vi "HOST.vi"() -> ()   [LabVIEW 2018]
uses:
  <vilib>/userdefined/High Color/nirio_resource_hc.ctl
  <vilib>/FPGAPlugInAG/PXI-7953R/niLvFpga_Open_PXI-7953R.vi
  <vilib>/rvi/interface/common/dynamic/niFpgaDynamicAddResources.vi
  <vilib>/FPGAPlugInAG/Dynamic/niLvFpga_Reset_Dynamic.vi
  <vilib>/FPGAPlugInAG/Dynamic/niLvFpga_Run_Dynamic.vi
  <vilib>/FPGAPlugInAG/PXI-7841R/niLvFpga_Open_PXI-7841R.vi
  <vilib>/Utility/error.llb/Error Cluster From Error Code.vi
  <vilib>/rvi/errors/niLvFpgaAdjustHostInterfaceError.vi
  <vilib>/rvi/interface/nirviOpenFPGA/nirviOpenFPGA.xnode
  FPGA Bitfiles/Testfor6581_FPGATarget_Testfor6581_omxlOdkNot8.lvbitx
  <vilib>/rvi/interface/nirviMethod/nirviMethod.xnode
  FPGA Bitfiles/Testfor65817841_FPGATarget2_Testfor7841_mCGf3KCUrBc.lvbitx
  <vilib>/rvi/interface/nirviReadWriteControl/nirviReadWriteControl.xnode
  NiFpgaLv.dll
  <vilib>/rvi/interface/Simulation/niFpgaSimulationCallBeginRW.vi
panel:
  in  "Connector0/DIO15":bool
  in  "Connector0/DIO14":bool
  in  "Connector0/DIO13":bool
  in  "Connector0/DIO12":bool
  in  "Connector0/DIO11":bool
  in  "Connector0/DIO10":bool
  in  "Connector0/DIO9":bool
  in  "Connector0/DIO8":bool
  in  "Connector0/DIO7":bool
  in  "Connector0/DIO6":bool
  in  "Connector0/DIO5":bool
  in  "Connector0/DIO4":bool
  in  "Connector1/DIO15":bool
  in  "Connector0/DIO3":bool
  in  "Connector0/DIO2":bool
  in  "Connector0/DIO1":bool
  in  "Connector0/DIO0":bool
  in  "Connector2/DIO0":bool
  in  "Connector2/DIO1":bool
  in  "Connector2/DIO2":bool
  in  "Connector2/DIO3":bool
  in  "Connector2/DIO4":bool
  in  "Connector2/DIO5":bool
  in  "Connector2/DIO6":bool
  in  "Connector2/DIO7":bool
  in  "Connector2/DIO8":bool
  in  "Connector2/DIO9":bool
  in  "Connector2/DIO10":bool
  in  "Connector2/DIO11":bool
  in  "Connector2/DIO12":bool
  in  "Connector2/DIO13":bool
  in  "Connector2/DIO14":bool
  in  "Connector2/DIO15":bool
  in  "Connector2/DIO16":bool
  in  "Connector2/DIO17":bool
  in  "Connector2/DIO18":bool
  in  "Connector2/DIO19":bool
  in  "Connector2/DIO20":bool
  in  "Connector2/DIO21":bool
  in  "Connector2/DIO22":bool
  in  "Connector2/DIO23":bool
  in  "Connector2/DIO24":bool
  in  "Connector2/DIO25":bool
  in  "Connector2/DIO26":bool
  in  "Connector2/DIO27":bool
  in  "Connector2/DIO28":bool
  in  "Connector2/DIO29":bool
  in  "Connector2/DIO30":bool
  in  "Connector2/DIO31":bool
  in  "Connector2/DIO32":bool
  in  "Connector2/DIO33":bool
  in  "Connector2/DIO34":bool
  in  "Connector2/DIO35":bool
  in  "Connector2/DIO36":bool
  in  "Connector2/DIO37":bool
  in  "Connector2/DIO38":bool
  in  "Connector2/DIO39":bool
  in  "Connector1/DIO39":bool
  in  "Connector1/DIO38":bool
  in  "Connector1/DIO37":bool
  in  "Connector1/DIO36":bool
  in  "Connector1/DIO35":bool
  in  "Connector1/DIO34":bool
  in  "Connector1/DIO33":bool
  in  "Connector1/DIO32":bool
  in  "Connector1/DIO31":bool
  in  "Connector1/DIO30":bool
  in  "Connector1/DIO29":bool
  in  "Connector1/DIO28":bool
  in  "Connector1/DIO27":bool
  in  "Connector1/DIO26":bool
  in  "Connector1/DIO25":bool
  in  "Connector1/DIO24":bool
  in  "Connector1/DIO23":bool
  in  "Connector1/DIO22":bool
  in  "Connector1/DIO21":bool
  in  "Connector1/DIO20":bool
  in  "Connector1/DIO19":bool
  in  "Connector1/DIO18":bool
  in  "Connector1/DIO17":bool
  in  "Connector1/DIO16":bool
  in  "Connector1/DIO14":bool
  in  "Connector1/DIO13":bool
  in  "Connector1/DIO12":bool
  in  "Connector1/DIO11":bool
  in  "Connector1/DIO10":bool
  in  "Connector1/DIO9":bool
  in  "Connector1/DIO8":bool
  in  "Connector1/DIO7":bool
  in  "Connector1/DIO6":bool
  in  "Connector1/DIO5":bool
  in  "Connector1/DIO4":bool
  in  "Connector1/DIO3":bool
  in  "Connector1/DIO2":bool
  in  "Connector1/DIO1":bool
  in  "Connector1/DIO0":bool
  out "Connector0/AI7":i16
  out "Connector0/AI6":i16
  out "Connector0/AI5":i16
  out "Connector0/AI4":i16
  out "Connector0/AI3":i16
  out "Connector0/AI2":i16
  out "Connector0/AI1":i16
  out "Connector0/AI0":i16
  in  "Connector0/AO7":i16
  in  "Connector0/AO6":i16
  in  "Connector0/AO5":i16
  in  "Connector0/AO4":i16
  in  "Connector0/AO3":i16
  in  "Connector0/AO2":i16
  in  "Connector0/AO1":i16
  in  "Connector0/AO0":i16
  in  "Tab Control":enum32{"7953", "7841"}(tab)
  in  "IO Module\\DDCA_DIO0_Write":bool
  in  "IO Module\\DDCA_DIO1_Write":bool
  in  "IO Module\\DDCA_DIO2_Write":bool
  in  "IO Module\\DDCA_DIO3_Write":bool
  in  "IO Module\\DDCA_DIO4_Write":bool
  in  "IO Module\\DDCA_DIO5_Write":bool
  in  "IO Module\\DDCA_DIO6_Write":bool
  in  "IO Module\\DDCA_DIO7_Write":bool
  in  "IO Module\\DDCA_DIO8_Write":bool
  in  "IO Module\\DDCA_DIO9_Write":bool
  in  "IO Module\\DDCA_DIO10_Write":bool
  in  "IO Module\\DDCA_DIO11_Write":bool
  in  "IO Module\\DDCA_DIO12_Write":bool
  in  "IO Module\\DDCA_DIO13_Write":bool
  in  "IO Module\\DDCA_DIO14_Write":bool
  in  "IO Module\\DDCA_DIO15_Write":bool
  in  "IO Module\\DDCA_DIO16_Write":bool
  in  "IO Module\\DDCA_DIO17_Write":bool
  in  "IO Module\\DDCA_DIO18_Write":bool
  in  "IO Module\\DDCA_DIO19_Write":bool
  in  "IO Module\\DDCA_DIO20_Write":bool
  in  "IO Module\\DDCA_DIO21_Write":bool
  in  "IO Module\\DDCA_DIO22_Write":bool
  in  "IO Module\\DDCA_DIO23_Write":bool
  in  "IO Module\\DDCA_PFI1_Write":bool
  in  "IO Module\\DDCA_PFI2_Write":bool
  in  "IO Module\\DDCA_PFI3_Write":bool
  in  "IO Module\\DDCB_DIO0_Write":bool
  in  "IO Module\\DDCB_DIO1_Write":bool
  in  "IO Module\\DDCB_DIO2_Write":bool
  in  "IO Module\\DDCB_DIO3_Write":bool
  in  "IO Module\\DDCB_DIO4_Write":bool
  in  "IO Module\\DDCB_DIO5_Write":bool
  in  "IO Module\\DDCB_DIO6_Write":bool
  in  "IO Module\\DDCB_DIO7_Write":bool
  in  "IO Module\\DDCB_DIO8_Write":bool
  in  "IO Module\\DDCB_DIO9_Write":bool
  in  "IO Module\\DDCB_DIO10_Write":bool
  in  "IO Module\\DDCB_DIO11_Write":bool
  in  "IO Module\\DDCB_DIO12_Write":bool
  in  "IO Module\\DDCB_DIO13_Write":bool
  in  "IO Module\\DDCB_DIO14_Write":bool
  in  "IO Module\\DDCB_DIO15_Write":bool
  in  "IO Module\\DDCB_DIO16_Write":bool
  in  "IO Module\\DDCB_DIO17_Write":bool
  in  "IO Module\\DDCB_DIO18_Write":bool
  in  "IO Module\\DDCB_DIO19_Write":bool
  in  "IO Module\\DDCB_DIO20_Write":bool
  in  "IO Module\\DDCB_DIO21_Write":bool
  in  "IO Module\\DDCB_DIO22_Write":bool
  in  "IO Module\\DDCB_DIO23_Write":bool
  in  "IO Module\\DDCB_PFI1_Write":bool
  in  "IO Module\\DDCB_PFI2_Write":bool
  in  "IO Module\\DDCB_PFI3_Write":bool
  in  "7841":T1="PXI1Slot6"
  in  "Devider Frequency 160/(x*2), x>0":u8=1 min=1
  in  "Constant(F) / Frequency(T)":bool
  in  "Стоп":bool
  in  "7953R":T1="PXI1Slot6"
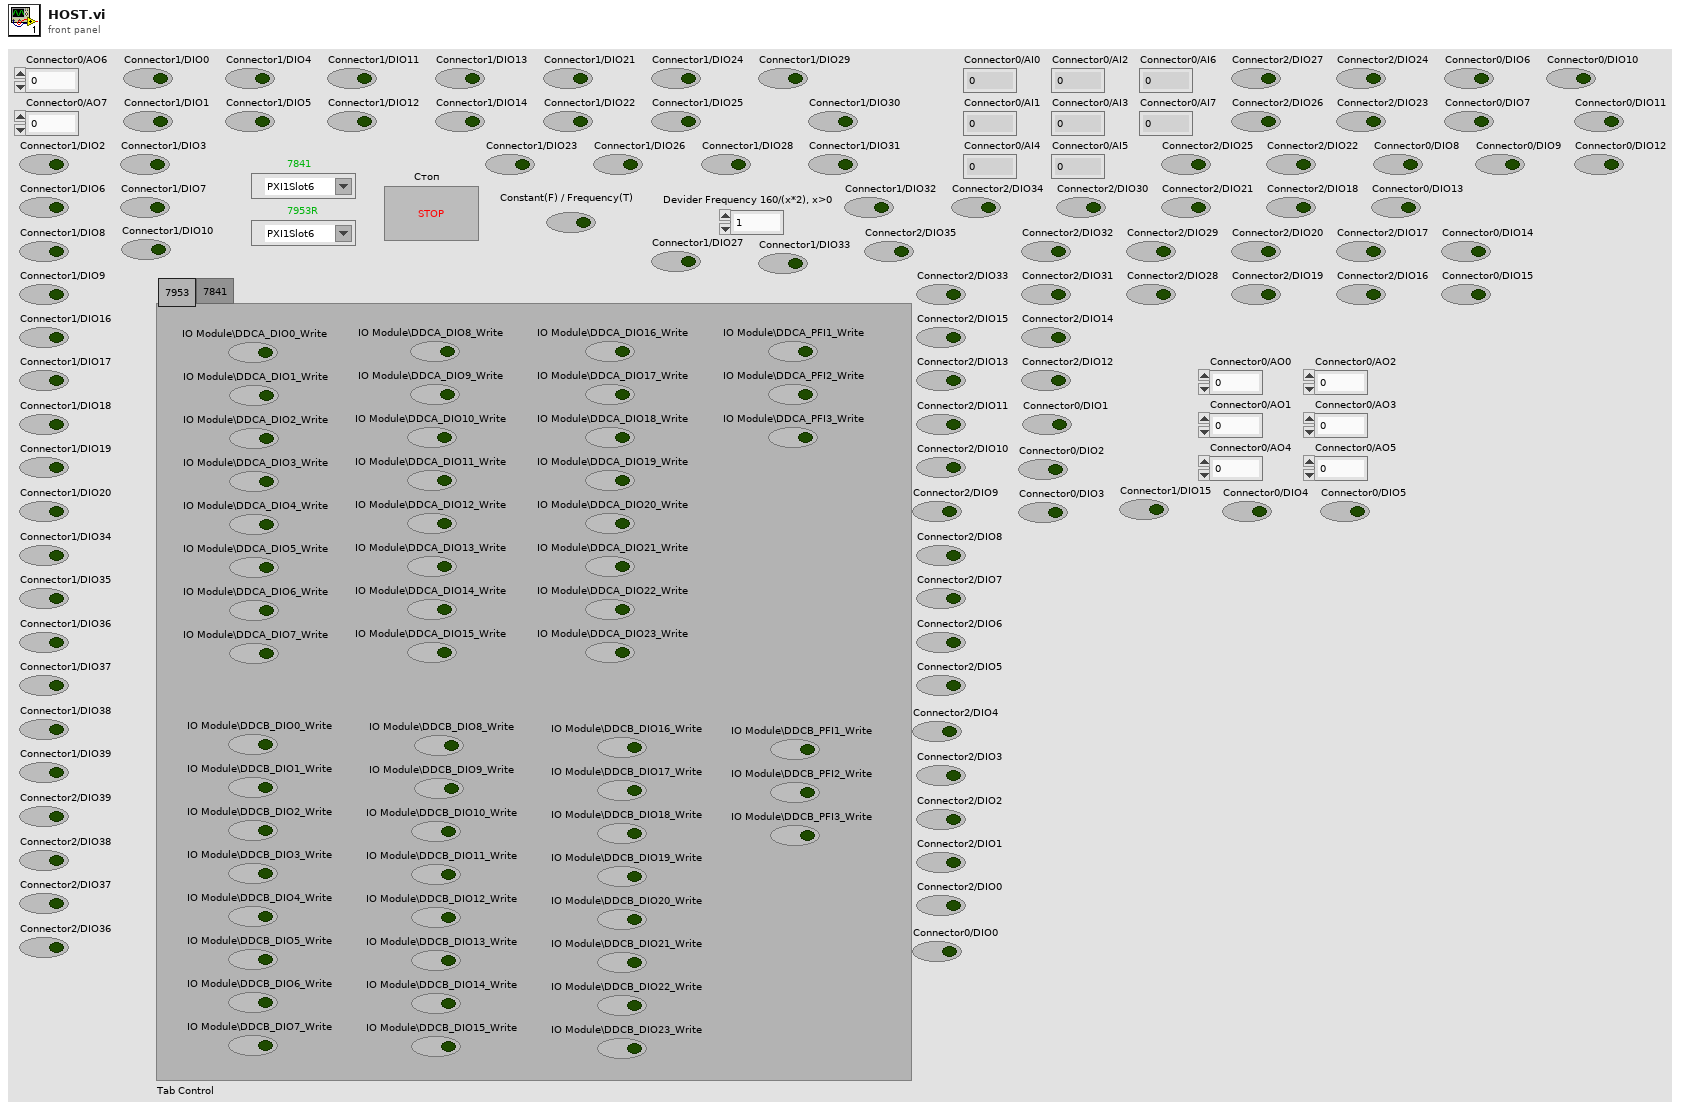
[diagram p1: front panel]
types:
  T1 = typedef "nirio_resource_hc.ctl" = tag
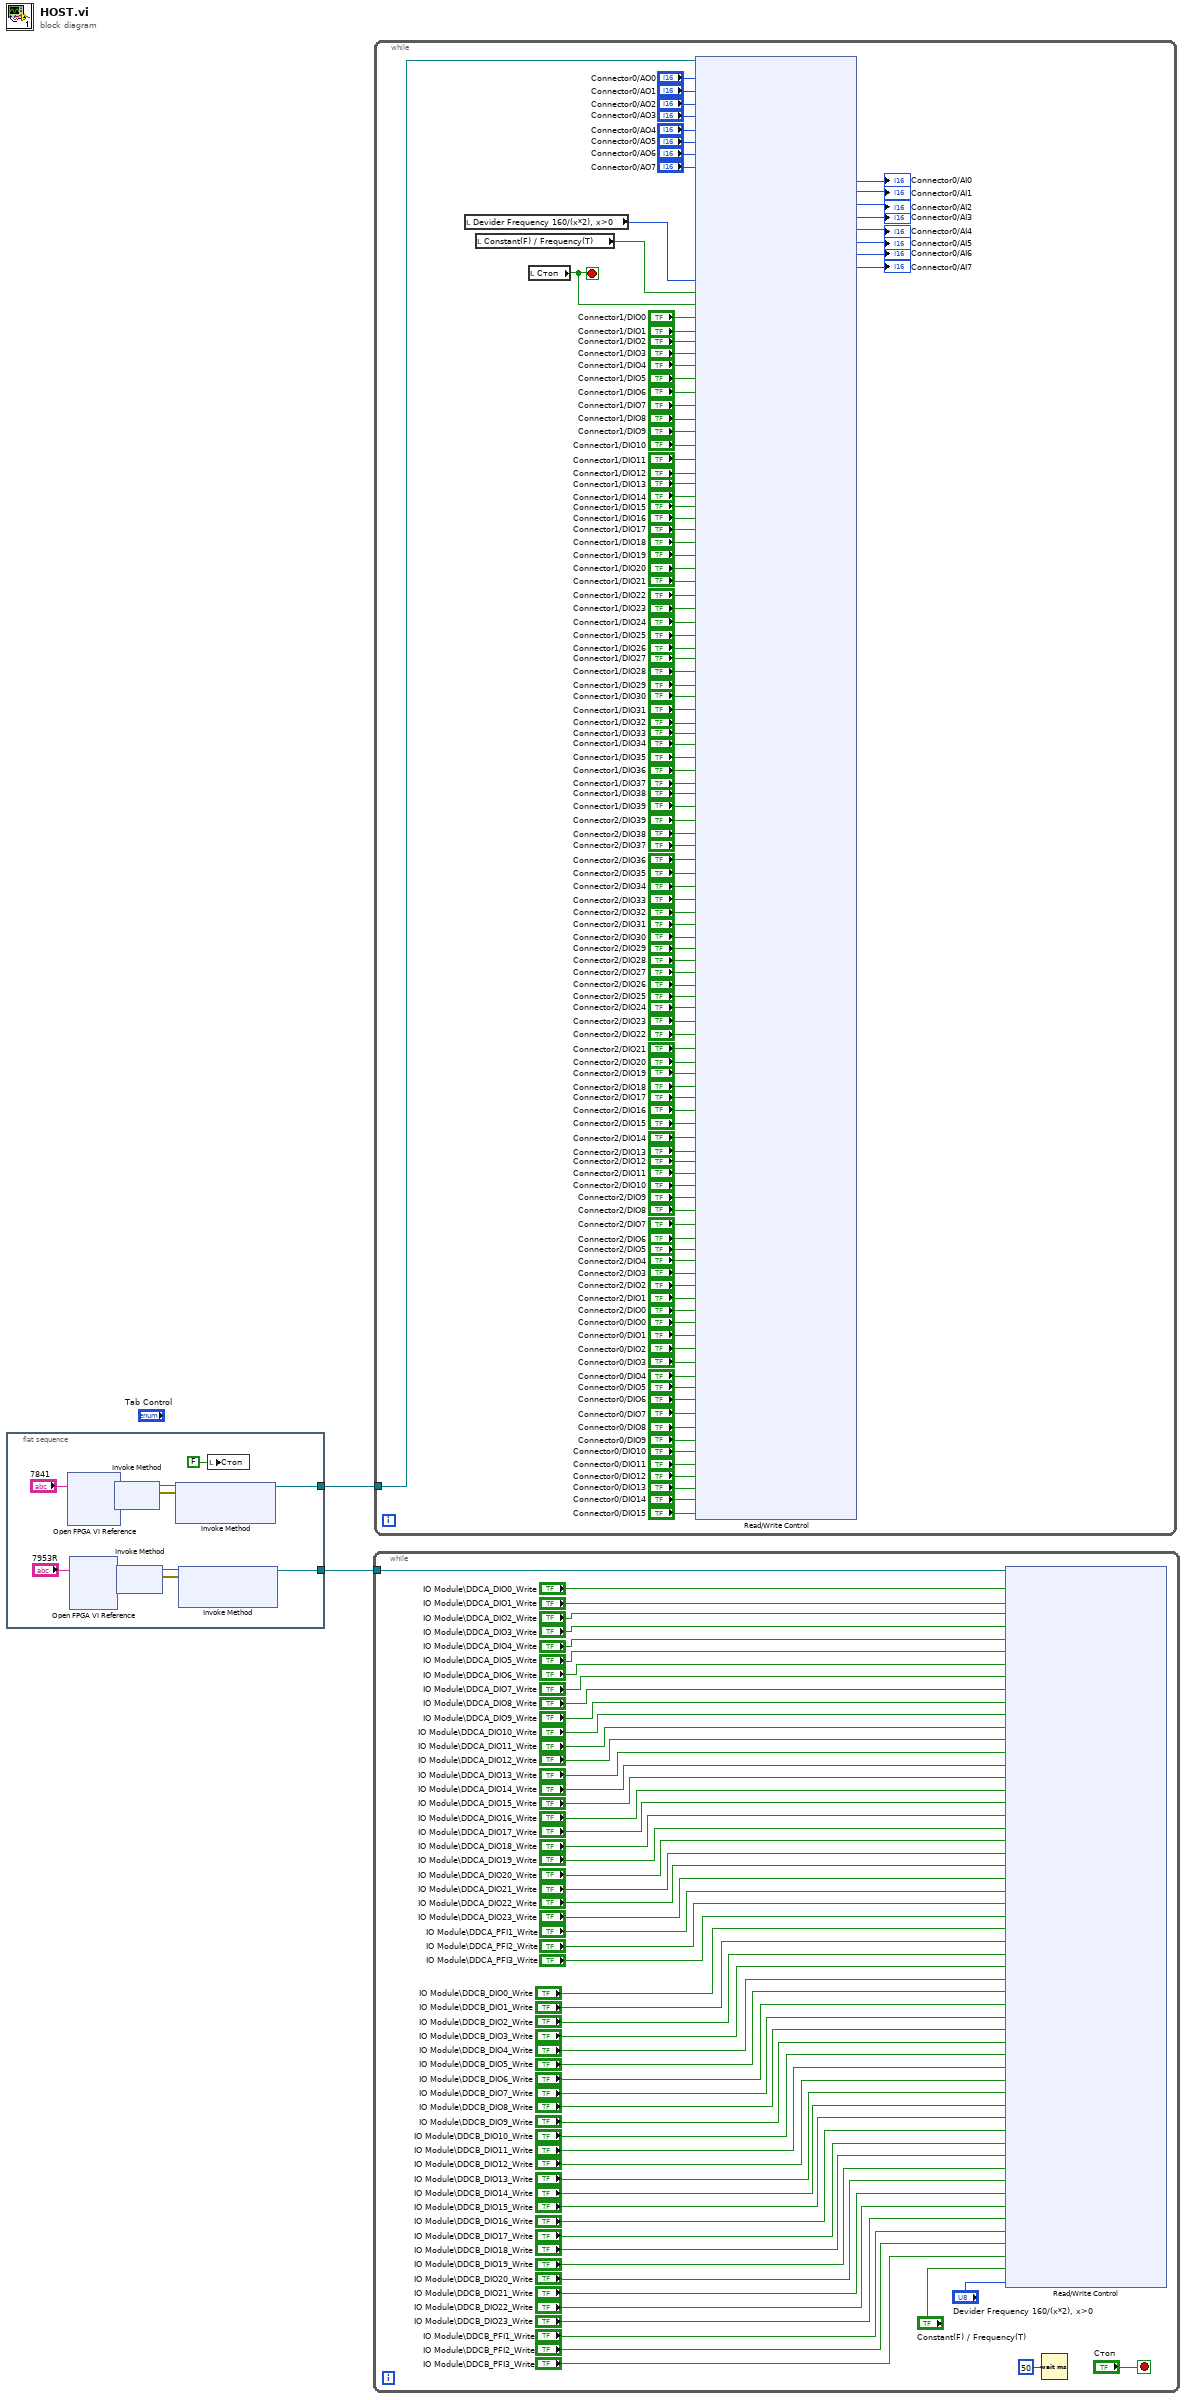
[diagram p0: block diagram]
diagram:
  n1 = flat-sequence {
    tunnel: [w10] -> w2
    tunnel: [w4] -> w1
    frame #0 {
      n2 = xnode "Open FPGA VI Reference"("resource name"="7841") -> ("FPGA VI Reference Out"=w9:refnum<k20>, "error out"=w7:errorcluster)  [unwired: 1 in]
      n3 = xnode "Open FPGA VI Reference"("resource name"="7953R") -> ("FPGA VI Reference Out"=w11:refnum<k20>, "error out"=w13:errorcluster)  [unwired: 1 in]
      n4 = xnode "Invoke Method"("FPGA VI Reference In"=w9, "error in"=w7) -> ("FPGA VI Reference Out"=w6:refnum<k20>, "error out"=w8:errorcluster)
      n5 = xnode "Invoke Method"("FPGA VI Reference In"=w11, "error in"=w13) -> ("FPGA VI Reference Out"=w14:refnum<k20>, "error out"=w12:errorcluster)
      n6 = xnode "Invoke Method"("FPGA VI Reference In"=w6, "error in"=w8) -> ("FPGA VI Reference Out"=w4:refnum<k20>)  [unwired: 1 in, 1 out]
      n7 = xnode "Invoke Method"("FPGA VI Reference In"=w14, "error in"=w12) -> ("FPGA VI Reference Out"=w10:refnum<k20>)  [unwired: 1 in, 1 out]
      n8 = local write "Стоп"(FALSE ("Стоп")) -> ()
    }
  }
  n9 = while {
    tunnel: w2 -> [w72]
    stop <- "Стоп" stop-if-true
    n10 = xnode "Read/Write Control"("FPGA VI Reference In"=w72, "IO Module\\DDCA_DIO0_Write"="IO Module\\DDCA_DIO0_Write", "IO Module\\DDCA_DIO1_Write"="IO Module\\DDCA_DIO1_Write", "IO Module\\DDCA_DIO2_Write"="IO Module\\DDCA_DIO2_Write", "IO Module\\DDCA_DIO3_Write"="IO Module\\DDCA_DIO3_Write", "IO Module\\DDCA_DIO4_Write"="IO Module\\DDCA_DIO4_Write", "IO Module\\DDCA_DIO5_Write"="IO Module\\DDCA_DIO5_Write", "IO Module\\DDCA_DIO6_Write"="IO Module\\DDCA_DIO6_Write", "IO Module\\DDCA_DIO7_Write"="IO Module\\DDCA_DIO7_Write", "IO Module\\DDCA_DIO8_Write"="IO Module\\DDCA_DIO8_Write", "IO Module\\DDCA_DIO9_Write"="IO Module\\DDCA_DIO9_Write", "IO Module\\DDCA_DIO10_Write"="IO Module\\DDCA_DIO10_Write", "IO Module\\DDCA_DIO11_Write"="IO Module\\DDCA_DIO11_Write", "IO Module\\DDCA_DIO12_Write"="IO Module\\DDCA_DIO12_Write", "IO Module\\DDCA_DIO13_Write"="IO Module\\DDCA_DIO13_Write", "IO Module\\DDCA_DIO14_Write"="IO Module\\DDCA_DIO14_Write", "IO Module\\DDCA_DIO15_Write"="IO Module\\DDCA_DIO15_Write", "IO Module\\DDCA_DIO16_Write"="IO Module\\DDCA_DIO16_Write", "IO Module\\DDCA_DIO17_Write"="IO Module\\DDCA_DIO17_Write", "IO Module\\DDCA_DIO18_Write"="IO Module\\DDCA_DIO18_Write", "IO Module\\DDCA_DIO19_Write"="IO Module\\DDCA_DIO19_Write", "IO Module\\DDCA_DIO20_Write"="IO Module\\DDCA_DIO20_Write", "IO Module\\DDCA_DIO21_Write"="IO Module\\DDCA_DIO21_Write", "IO Module\\DDCA_DIO22_Write"="IO Module\\DDCA_DIO22_Write", "IO Module\\DDCA_DIO23_Write"="IO Module\\DDCA_DIO23_Write", "IO Module\\DDCA_PFI1_Write"="IO Module\\DDCA_PFI1_Write", "IO Module\\DDCA_PFI2_Write"="IO Module\\DDCA_PFI2_Write", "IO Module\\DDCA_PFI3_Write"="IO Module\\DDCA_PFI3_Write", "IO Module\\DDCB_DIO0_Write"="IO Module\\DDCB_DIO0_Write", "IO Module\\DDCB_DIO1_Write"="IO Module\\DDCB_DIO1_Write", "IO Module\\DDCB_DIO2_Write"="IO Module\\DDCB_DIO2_Write", "IO Module\\DDCB_DIO3_Write"="IO Module\\DDCB_DIO3_Write", "IO Module\\DDCB_DIO4_Write"="IO Module\\DDCB_DIO4_Write", "IO Module\\DDCB_DIO5_Write"="IO Module\\DDCB_DIO5_Write", "IO Module\\DDCB_DIO6_Write"="IO Module\\DDCB_DIO6_Write", "IO Module\\DDCB_DIO7_Write"="IO Module\\DDCB_DIO7_Write", "IO Module\\DDCB_DIO8_Write"="IO Module\\DDCB_DIO8_Write", "IO Module\\DDCB_DIO9_Write"="IO Module\\DDCB_DIO9_Write", "IO Module\\DDCB_DIO10_Write"="IO Module\\DDCB_DIO10_Write", "IO Module\\DDCB_DIO11_Write"="IO Module\\DDCB_DIO11_Write", "IO Module\\DDCB_DIO12_Write"="IO Module\\DDCB_DIO12_Write", "IO Module\\DDCB_DIO13_Write"="IO Module\\DDCB_DIO13_Write", "IO Module\\DDCB_DIO14_Write"="IO Module\\DDCB_DIO14_Write", "IO Module\\DDCB_DIO15_Write"="IO Module\\DDCB_DIO15_Write", "IO Module\\DDCB_DIO16_Write"="IO Module\\DDCB_DIO16_Write", "IO Module\\DDCB_DIO17_Write"="IO Module\\DDCB_DIO17_Write", "IO Module\\DDCB_DIO18_Write"="IO Module\\DDCB_DIO18_Write", "IO Module\\DDCB_DIO19_Write"="IO Module\\DDCB_DIO19_Write", "IO Module\\DDCB_DIO20_Write"="IO Module\\DDCB_DIO20_Write", "IO Module\\DDCB_DIO21_Write"="IO Module\\DDCB_DIO21_Write", "IO Module\\DDCB_DIO22_Write"="IO Module\\DDCB_DIO22_Write", "IO Module\\DDCB_DIO23_Write"="IO Module\\DDCB_DIO23_Write", "IO Module\\DDCB_PFI1_Write"="IO Module\\DDCB_PFI1_Write", "IO Module\\DDCB_PFI2_Write"="IO Module\\DDCB_PFI2_Write", "IO Module\\DDCB_PFI3_Write"="IO Module\\DDCB_PFI3_Write", "Constant(F) / Frequency(T)"="Constant(F) / Frequency(T)", "Devider Frequency 160/(x*2), x>0"="Devider Frequency 160/(x*2), x>0") -> ()  [unwired: 1 in, 2 out]
    n11 = Wait (ms)(milliseconds to wait=u32 50) -> ()  [unwired: 1 out]
  }
  n12 = while {
    tunnel: w1 -> [w190]
    stop <- w171 stop-if-true
    n13 = local read "Devider Frequency 160/(x*2), x>0"() -> (w189:u8)
    n14 = local read "Constant(F) / Frequency(T)"() -> (w188:bool)
    n15 = local read "Стоп"() -> (w171:bool)
    n16 = xnode "Read/Write Control"("FPGA VI Reference In"=w190, "Connector0/AO0"="Connector0/AO0", "Connector0/AO1"="Connector0/AO1", "Connector0/AO2"="Connector0/AO2", "Connector0/AO3"="Connector0/AO3", "Connector0/AO4"="Connector0/AO4", "Connector0/AO5"="Connector0/AO5", "Connector0/AO6"="Connector0/AO6", "Connector0/AO7"="Connector0/AO7", "Devider Frequency 160/(x*2), x>0"=w189, "Constant(F) / Frequency(T)"=w188, "Стоп"=w171, "Connector1/DIO0"="Connector1/DIO0", "Connector1/DIO1"="Connector1/DIO1", "Connector1/DIO2"="Connector1/DIO2", "Connector1/DIO3"="Connector1/DIO3", "Connector1/DIO4"="Connector1/DIO4", "Connector1/DIO5"="Connector1/DIO5", "Connector1/DIO6"="Connector1/DIO6", "Connector1/DIO7"="Connector1/DIO7", "Connector1/DIO8"="Connector1/DIO8", "Connector1/DIO9"="Connector1/DIO9", "Connector1/DIO10"="Connector1/DIO10", "Connector1/DIO11"="Connector1/DIO11", "Connector1/DIO12"="Connector1/DIO12", "Connector1/DIO13"="Connector1/DIO13", "Connector1/DIO14"="Connector1/DIO14", "Connector1/DIO15"="Connector1/DIO15", "Connector1/DIO16"="Connector1/DIO16", "Connector1/DIO17"="Connector1/DIO17", "Connector1/DIO18"="Connector1/DIO18", "Connector1/DIO19"="Connector1/DIO19", "Connector1/DIO20"="Connector1/DIO20", "Connector1/DIO21"="Connector1/DIO21", "Connector1/DIO22"="Connector1/DIO22", "Connector1/DIO23"="Connector1/DIO23", "Connector1/DIO24"="Connector1/DIO24", "Connector1/DIO25"="Connector1/DIO25", "Connector1/DIO26"="Connector1/DIO26", "Connector1/DIO27"="Connector1/DIO27", "Connector1/DIO28"="Connector1/DIO28", "Connector1/DIO29"="Connector1/DIO29", "Connector1/DIO30"="Connector1/DIO30", "Connector1/DIO31"="Connector1/DIO31", "Connector1/DIO32"="Connector1/DIO32", "Connector1/DIO33"="Connector1/DIO33", "Connector1/DIO34"="Connector1/DIO34", "Connector1/DIO35"="Connector1/DIO35", "Connector1/DIO36"="Connector1/DIO36", "Connector1/DIO37"="Connector1/DIO37", "Connector1/DIO38"="Connector1/DIO38", "Connector1/DIO39"="Connector1/DIO39", "Connector2/DIO39"="Connector2/DIO39", "Connector2/DIO38"="Connector2/DIO38", "Connector2/DIO37"="Connector2/DIO37", "Connector2/DIO36"="Connector2/DIO36", "Connector2/DIO35"="Connector2/DIO35", "Connector2/DIO34"="Connector2/DIO34", "Connector2/DIO33"="Connector2/DIO33", "Connector2/DIO32"="Connector2/DIO32", "Connector2/DIO31"="Connector2/DIO31", "Connector2/DIO30"="Connector2/DIO30", "Connector2/DIO29"="Connector2/DIO29", "Connector2/DIO28"="Connector2/DIO28", "Connector2/DIO27"="Connector2/DIO27", "Connector2/DIO26"="Connector2/DIO26", "Connector2/DIO25"="Connector2/DIO25", "Connector2/DIO24"="Connector2/DIO24", "Connector2/DIO23"="Connector2/DIO23", "Connector2/DIO22"="Connector2/DIO22", "Connector2/DIO21"="Connector2/DIO21", "Connector2/DIO20"="Connector2/DIO20", "Connector2/DIO19"="Connector2/DIO19", "Connector2/DIO18"="Connector2/DIO18", "Connector2/DIO17"="Connector2/DIO17", "Connector2/DIO16"="Connector2/DIO16", "Connector2/DIO15"="Connector2/DIO15", "Connector2/DIO14"="Connector2/DIO14", "Connector2/DIO13"="Connector2/DIO13", "Connector2/DIO12"="Connector2/DIO12", "Connector2/DIO11"="Connector2/DIO11", "Connector2/DIO10"="Connector2/DIO10", "Connector2/DIO9"="Connector2/DIO9", "Connector2/DIO8"="Connector2/DIO8", "Connector2/DIO7"="Connector2/DIO7", "Connector2/DIO6"="Connector2/DIO6", "Connector2/DIO5"="Connector2/DIO5", "Connector2/DIO4"="Connector2/DIO4", "Connector2/DIO3"="Connector2/DIO3", "Connector2/DIO2"="Connector2/DIO2", "Connector2/DIO1"="Connector2/DIO1", "Connector2/DIO0"="Connector2/DIO0", "Connector0/DIO0"="Connector0/DIO0", "Connector0/DIO1"="Connector0/DIO1", "Connector0/DIO2"="Connector0/DIO2", "Connector0/DIO3"="Connector0/DIO3", "Connector0/DIO4"="Connector0/DIO4", "Connector0/DIO5"="Connector0/DIO5", "Connector0/DIO6"="Connector0/DIO6", "Connector0/DIO7"="Connector0/DIO7", "Connector0/DIO8"="Connector0/DIO8", "Connector0/DIO9"="Connector0/DIO9", "Connector0/DIO10"="Connector0/DIO10", "Connector0/DIO11"="Connector0/DIO11", "Connector0/DIO12"="Connector0/DIO12", "Connector0/DIO13"="Connector0/DIO13", "Connector0/DIO14"="Connector0/DIO14", "Connector0/DIO15"="Connector0/DIO15") -> ("Connector0/AI0"=→"Connector0/AI0":i16, "Connector0/AI1"=→"Connector0/AI1":i16, "Connector0/AI2"=→"Connector0/AI2":i16, "Connector0/AI3"=→"Connector0/AI3":i16, "Connector0/AI4"=→"Connector0/AI4":i16, "Connector0/AI5"=→"Connector0/AI5":i16, "Connector0/AI6"=→"Connector0/AI6":i16, "Connector0/AI7"=→"Connector0/AI7":i16)  [unwired: 1 in, 2 out]
  }
